vi "provide input data to library.vi"(8 "error in":errorcluster, 10 "data in":string, 11 "lvsocket":u64) -> (0 "error out":errorcluster, 3 "return":i32)   [LabVIEW 2016, in "lv tls dll.lvlib"]
uses:
  lv tls dll.lvlib
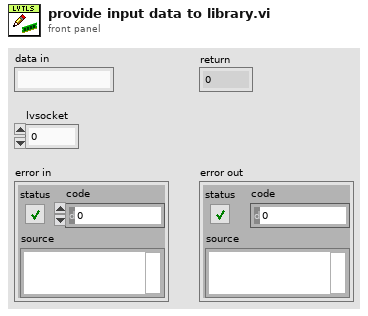
[diagram p1: front panel]
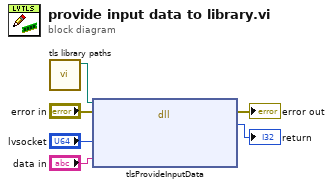
[diagram p0: block diagram]
diagram:
  n1 = call "tls library paths.vi"() -> ("lvtls"=w6:path)  [unwired: 8 in, 3 out]
  n2 = dll-call lib="C:/Users/IEUser/Desktop/tlssimple/lvlibtls.dll" fn="tlsProvideInputData"(path in=w6, error in="error in", "lvsocket"="lvsocket", "data"="data in") -> (error out=→"error out":errorcluster, "err"=→"return":i32)  [unwired: 3 in, 1 out]
